vi "#182_MAV_MSG_AHRS3_DECODE.vi"(11 "mavlink_payload":u8[](array[numeric])) -> (3 "AHRS3":T1)   [LabVIEW 2023]
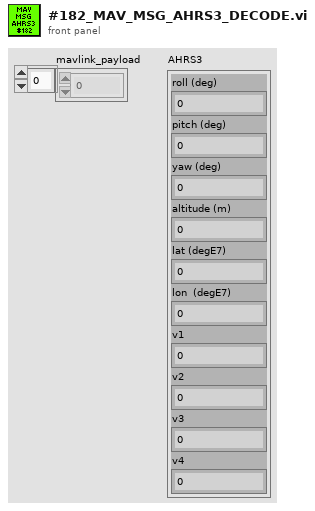
[diagram p1: front panel]
types:
  T1 = cluster{"roll (deg)":sgl, "pitch (deg)":sgl, "yaw (deg)":sgl, "altitude (m)":sgl, "lat (degE7)":i32, "lon  (degE7)":i32, "v1":sgl, "v2":sgl, "v3":sgl, "v4":sgl}
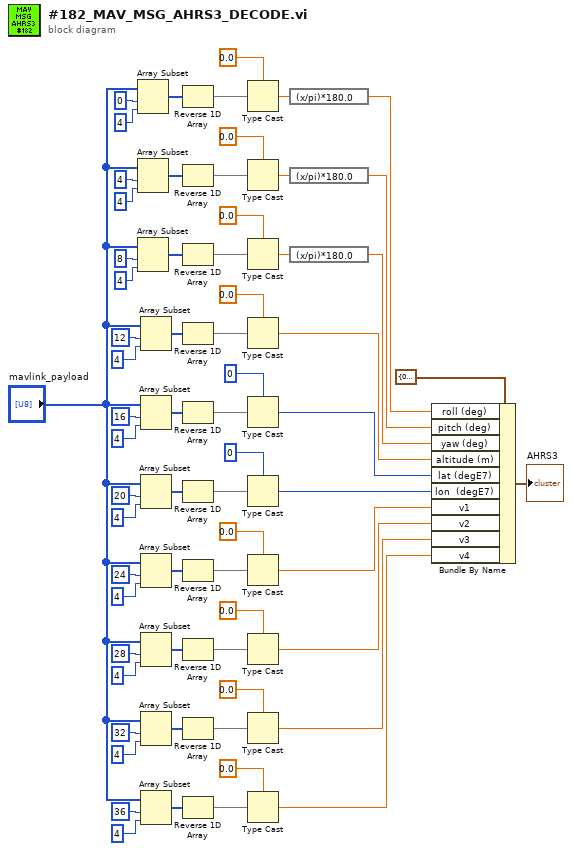
[diagram p0: block diagram]
diagram:
  n1 = Array Subset(array="mavlink_payload", index=0 ("Index"), length=4) -> (w65:u8[])
  n2 = Array Subset(array="mavlink_payload", index=4 ("Index"), length=4) -> (w58:u8[])
  n3 = Array Subset(array="mavlink_payload", index=8 ("Index"), length=4) -> (w51:u8[])
  n4 = Array Subset(array="mavlink_payload", index=12 ("Index"), length=4) -> (w44:u8[])
  n5 = Array Subset(array="mavlink_payload", index=16 ("Index"), length=4) -> (w38:u8[])
  n6 = Array Subset(array="mavlink_payload", index=20 ("Index"), length=4) -> (w32:u8[])
  n7 = Array Subset(array="mavlink_payload", index=24 ("Index"), length=4) -> (w26:u8[])
  n8 = Array Subset(array="mavlink_payload", index=28 ("Index"), length=4) -> (w18:u8[])
  n9 = Array Subset(array="mavlink_payload", index=32 ("Index"), length=4) -> (w12:u8[])
  n10 = Array Subset(array="mavlink_payload", index=36 ("Index"), length=4) -> (w6:u8[])
  n11 = Reverse 1D Array(array=w65) -> (reversed array=w64:u8[])
  n12 = Reverse 1D Array(array=w58) -> (reversed array=w57:u8[])
  n13 = Reverse 1D Array(array=w51) -> (reversed array=w50:u8[])
  n14 = Reverse 1D Array(array=w44) -> (reversed array=w43:u8[])
  n15 = Reverse 1D Array(array=w38) -> (reversed array=w37:u8[])
  n16 = Reverse 1D Array(array=w32) -> (reversed array=w31:u8[])
  n17 = Reverse 1D Array(array=w26) -> (reversed array=w25:u8[])
  n18 = Reverse 1D Array(array=w18) -> (reversed array=w17:u8[])
  n19 = Reverse 1D Array(array=w12) -> (reversed array=w11:u8[])
  n20 = Reverse 1D Array(array=w6) -> (reversed array=w5:u8[])
  n21 = Type Cast(type=sgl 0.0 ("Index"), x=w64) -> (*(type *) &x=w61:sgl)
  n22 = Type Cast(type=sgl 0.0 ("Index"), x=w57) -> (*(type *) &x=w54:sgl)
  n23 = Type Cast(type=sgl 0.0 ("Index"), x=w50) -> (*(type *) &x=w47:sgl)
  n24 = Type Cast(type=sgl 0.0 ("Index"), x=w43) -> (*(type *) &x=w40:sgl)
  n25 = Type Cast(type=0 ("Index"), x=w37) -> (*(type *) &x=w34:i32)
  n26 = Type Cast(type=0 ("Index"), x=w31) -> (*(type *) &x=w28:i32)
  n27 = Type Cast(type=sgl 0.0 ("Index"), x=w25) -> (*(type *) &x=w22:sgl)
  n28 = Type Cast(type=sgl 0.0 ("Index"), x=w17) -> (*(type *) &x=w14:sgl)
  n29 = Type Cast(type=sgl 0.0 ("Index"), x=w11) -> (*(type *) &x=w8:sgl)
  n30 = Type Cast(type=sgl 0.0 ("Index"), x=w5) -> (*(type *) &x=w1:sgl)
  n31 = expression code="(x/pi)*180.0" ("radians to degrees")(w61) -> (w60:sgl)
  n32 = expression code="(x/pi)*180.0" ("radians to degrees")(w54) -> (w53:sgl)
  n33 = expression code="(x/pi)*180.0" ("radians to degrees")(w47) -> (w46:sgl)
  n34 = Bundle By Name(cluster=T1 {"roll (deg)"=0.0, "pitch (deg)"=0.0, "yaw (deg)"=0.0, "altitude (m)"=0.0, "lat (degE7)"=0, "lon  (degE7)"=0, "v1"=0.0, "v2"=0.0, "v3"=0.0, "v4"=0.0} ("AHRS3"), "roll (deg)"=w60, "pitch (deg)"=w53, "yaw (deg)"=w46, "altitude (m)"=w40, "lat (degE7)"=w34, "lon  (degE7)"=w28, "v1"=w22, "v2"=w14, "v3"=w8, "v4"=w1) -> (→"AHRS3":T1)
